vi "WM_CAP - To fourcc.vi"(7 "biCompression":i32 format="%.0x") -> (8 "FOURCC":string)   [LabVIEW 2022 SP3]
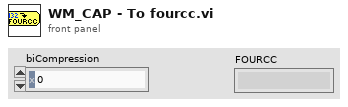
[diagram p1: front panel]
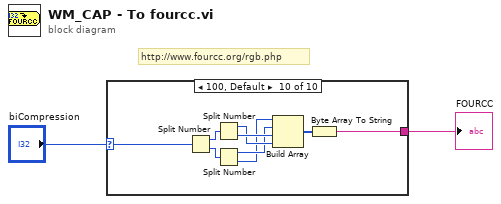
[diagram p0: block diagram]
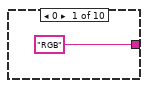
[diagram p2: hidden frame]
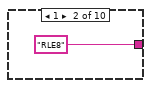
[diagram p3: hidden frame]
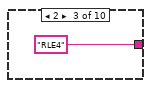
[diagram p4: hidden frame]
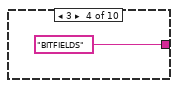
[diagram p5: hidden frame]
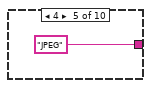
[diagram p6: hidden frame]
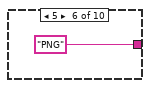
[diagram p7: hidden frame]
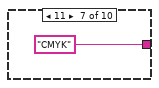
[diagram p8: hidden frame]
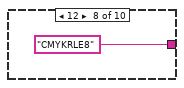
[diagram p9: hidden frame]
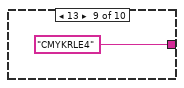
[diagram p10: hidden frame]
diagram:
  # "http://www.fourcc.org/rgb.php"
  n1 = case shown="100, Default" "biCompression" {
    selector: "biCompression" -> [_ _ _ _ _ _ _ _ _ w12]
    tunnel: ["RGB" ("string") "RLE8" ("string") "RLE4" ("string") "BITFIELDS" ("string") "JPEG" ("string") "PNG" ("string") "CMYK" ("string") "CMYKRLE8" ("string") "CMYKRLE4" ("string") w17] -> w1
    frame 0 {
    }
    frame 1 {
    }
    frame 2 {
    }
    frame 3 {
    }
    frame 4 {
    }
    frame 5 {
    }
    frame 11 {
    }
    frame 12 {
    }
    frame 13 {
    }
    frame 100, Default {
      n2 = Split Number(x=w12) -> (hi(x)=w20:u16, lo(x)=w19:u16)
      n3 = Split Number(x=w20) -> (hi(x)=w15:u8, lo(x)=w16:u8)
      n4 = Split Number(x=w19) -> (hi(x)=w14:u8, lo(x)=w13:u8)
      n5 = Build Array(w13, w14, w16, w15) -> (w18:u8[])
      n6 = Byte Array To String(unsigned byte array=w18) -> (string=w17:string)
    }
  }
  "FOURCC" <- w1
